vi "Create WAMP msg.vi"(8 "error in (no error)":errorcluster, 11 "Realm":string) -> (0 "error out":errorcluster, 3 "WAMP message":string)   [LabVIEW 2021, in "wamplv.lvlib" / "WAMP Client.lvclass"]
uses:
  WAMP Client.lvclass
  WAMP Client.lvclass/WAMP Client.ctl
  TypeDef/WAMP Message Codes.ctl
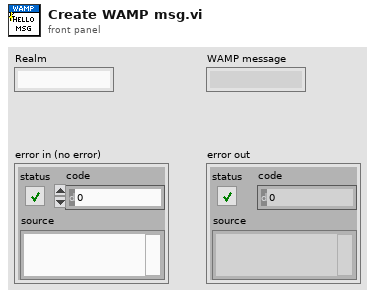
[diagram p1: front panel]
types:
  T1 = typedef "wamplv.lvlib/WAMP Client.lvclass/WAMP Message Codes.ctl" = u16
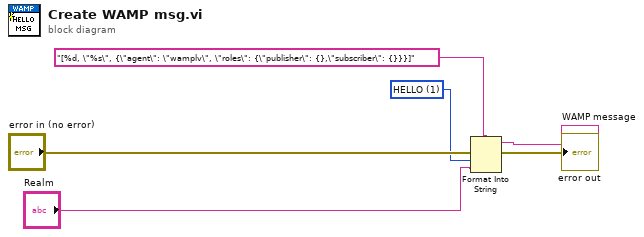
[diagram p0: block diagram]
diagram:
  w1 = T1 1 items=["HELLO"=1, "WELCOME"=2, "ABORT"=3, "GOODBYE"=6, "ERROR"=8, "PUBLISH"=16, "PUBLISHED"=17, "SUBSCRIBE"=32, "SUBSCRIBED"=33, "UNSUBSCRIBE"=34, "UNSUBSCRIBED"=35, "EVENT"=36, "CALL"=48, "RESULT"=59, "REGISTER"=64, "REGISTERED"=65, "UNREGISTER"=66, "UNREGISTERED"=67, "INVOCATION"=68, "YIELD"=70] ("Message Codes")
  n1 = Format Into String(format string="[%d, \"%s\", {\"agent\": \"wamplv\", \"roles\": {\"publisher\": {},\"subscriber\": {}}}]", error in="error in (no error)", w1, "Realm") -> (resulting string=→"WAMP message":string, error out=→"error out":errorcluster)  [unwired: 1 in]
